vi "WorkorderHandler_NotAReference.vi"(1 "reference":T1) -> (0 "not a reference?":bool)   [LabVIEW 2011]
doc: "Returns TRUE if dqGOOP object refnum is not a refnum. Otherwise, this function returns FALSE. Use this function to make sure a refnum to a dqGOOP object still resides in system memory and was not closed."
uses:
  DataStructures/WorkorderHandler_ObjectReference.ctl
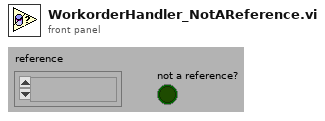
[diagram p1: front panel]
types:
  T1 = typedef "WorkorderHandler_ObjectReference.ctl" = refnum<k1>
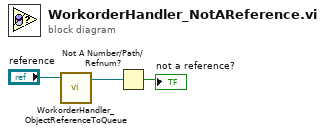
[diagram p0: block diagram]
diagram:
  n1 = call "WorkorderHandler_ObjectReferenceToQueue.vi"("reference"="reference") -> ("queue"=w2:refnum<queue>)  [unwired: 26 out]
  n2 = Not A Number/Path/Refnum?(number/path/refnum=w2) -> (NaN/Path/Refnum?=→"not a reference?":bool)
